vi "Tracer_Level__VIStart.vi"(11 "Calltree Level":i32) -> (2 "Trace Enabled":bool, 3 "Category":string)   [LabVIEW 2018, in "TracerLibrary.lvlib" / "Tracer.lvclass"]
uses:
  Tracer.lvclass
  protected/Tracer_ClassAttributes.vi
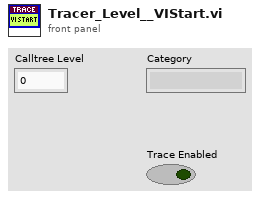
[diagram p1: front panel]
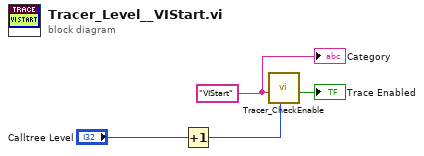
[diagram p0: block diagram]
diagram:
  w4 = "VIStart" ("Category")
  n1 = Increment(x="Calltree Level") -> (x+1=w1:i32)
  n2 = call "Tracer_CheckEnable.vi"("Calltree Level"=w1, "Category"=w4) -> ("Trace Enabled"=→"Trace Enabled":bool)  [unwired: 9 in]
  "Category" <- w4
